vi "Write Drive from Slot.vi"(8 "error in":errorcluster, 10 "drive from slot":T1, 11 "counter driven output mode in":refnum<class "Counter Driven Output Mode.lvclass">) -> (0 "error out":errorcluster, 3 "counter driven output mode out":refnum<class "Counter Driven Output Mode.lvclass">)   [LabVIEW 2020, in "Scan Engine Scripting.lvlib" / "Counter Driven Output Mode.lvclass"]
uses:
  Counter Driven Output Mode.lvclass
  Drive from Slot.ctl
  Counter Driven Output Mode.lvclass/Counter Driven Output Mode.ctl
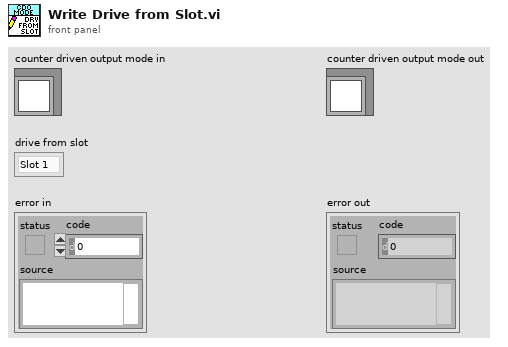
[diagram p1: front panel]
types:
  T1 = typedef "Scan Engine Scripting.lvlib/Counter Driven Output Mode.lvclass/Drive from Slot.ctl" = enum16{"Slot 1", "Slot 2", "Slot 3", "Slot 4", "Slot 5", "Slot 6", "Slot 7", "Slot 8"}
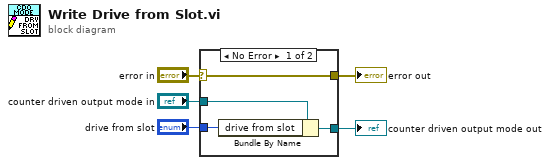
[diagram p0: block diagram]
diagram:
  n1 = case shown="No Error" "error in" {
    selector: "error in" -> [w9 w10]
    tunnel: [w9 w10] -> w4
    tunnel: [w7 w11] -> w2
    tunnel: "counter driven output mode in" -> [w8 w11]
    tunnel: "drive from slot" -> [w6 _]
    frame No Error {
      n2 = Bundle By Name(cluster=w8, "drive from slot"=w6) -> (w7:refnum<class "Counter Driven Output Mode.lvclass">)
    }
    frame Error {
    }
  }
  "error out" <- w4
  "counter driven output mode out" <- w2
